vi "filter.vi"() -> ()   [LabVIEW 2018]
uses:
  <vilib>/Instr/_visa.llb/VISA Configure Serial Port (Instr).vi
panel:
  out "error out":errorcluster
  in  "stop":bool
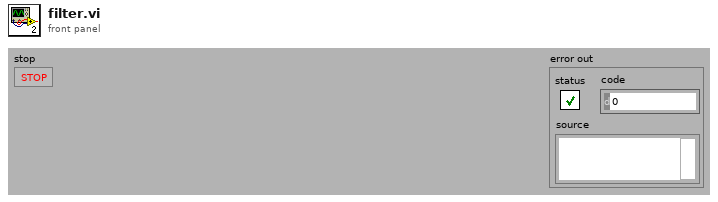
[diagram p1: front panel]
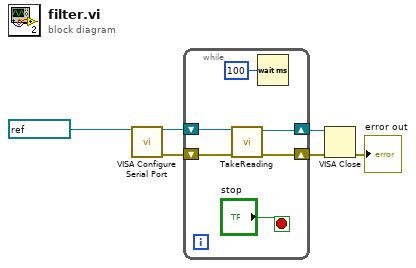
[diagram p0: block diagram]
diagram:
  n1 = call-poly "VISA Configure Serial Port"("VISA resource name"=refnum<visa-resource-name> "COM6") -> ("VISA resource name out"=w5:refnum<visa-resource-name>, "error out"=w3:errorcluster)  [unwired: 13 in]
  n2 = while {
    shift-right: [w10] -> w4
    shift-left: w5 -> [w11]
    shift-right: [w8] -> w2
    shift-left: w3 -> [w9]
    stop <- "stop" stop-if-true
    n3 = call "TakeReading.vi"("error in"=w9, "Port"=w11) -> ("error out"=w8:errorcluster, "Port out"=w10:refnum<visa-resource-name>)  [unwired: 6 in, 2 out]
    n4 = Wait (ms)(milliseconds to wait=u32 100) -> ()  [unwired: 1 out]
  }
  n5 = VISA Close(VISA resource name=w4, error in (no error)=w2) -> (error out=→"error out":errorcluster)
